vi "DSF.Engine.Execution.Builder.Initialize Intermediate Buffers.vi"(8 "error in (no error)":errorcluster, 11 "Builder in":refnum<class "DSF.Engine.Execution.Builder.lvclass">) -> (0 "error out":errorcluster, 2 "Data Type Buffers":T1, 3 "Builder out":refnum<class "DSF.Engine.Execution.Builder.lvclass">)   [LabVIEW 2016, in "DSF.Engine.lvlib" / "DSF.Engine.Execution.Builder.lvclass"]
uses:
  DSF.Engine.Execution.Builder.lvclass
  DSF.Engine.Execution.Builder.Type Buffers.ctl
  DSF.Engine.Execution.Builder.lvclass/DSF.Engine.Execution.Builder.ctl
  Cache/DSF.Engine.Memory.Cache.Framework.lvclass/DSF.Engine.Memory.Cache.Framework.ctl
  Cache/DSF.Engine.Memory.Cache.Plugin.lvclass/DSF.Engine.Memory.Cache.Plugin.ctl
  Cache/DSF.Engine.Memory.Cache.Transfer.lvclass/DSF.Engine.Memory.Cache.Transfer.ctl
  Cache/DSF.Engine.Memory.Cache.Framework.Get Plugin Caches.vi
  Cache/DSF.Engine.Memory.Cache.Plugin.Get Largest Count.All Types.vi
  Cache/DSF.Engine.Memory.Cache.Plugin.Get Transfer Caches.vi
  Cache/DSF.Engine.Memory.Cache.Transfer.Get Largest Count.All Types.vi
  Cache/DSF.Engine.Memory.Cache.Transfer.Get Channel Configuration.vi
  Cache/DSF.Engine.Memory.Cache.Framework.lvclass
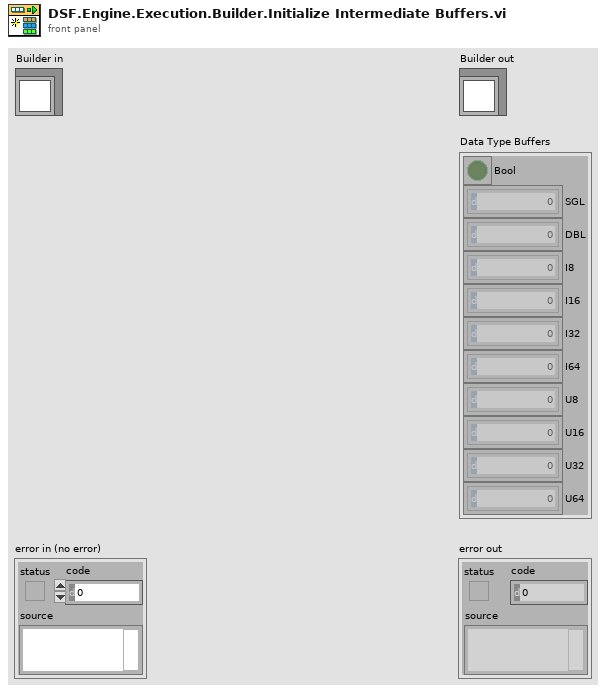
[diagram p1: front panel]
types:
  T1 = typedef "DSF.Engine.lvlib/DSF.Engine.Execution.Builder.lvclass/DSF.Engine.Execution.Builder.Type Buffers.ctl" = cluster{"Bool":bool[], "SGL":sgl[], "DBL":dbl[], "I8":i8[], "I16":i16[], "I32":i32[], "I64":i64[], "U8":u8[], "U16":u16[], "U32":u32[], "U64":u64[]}
  T2 = typedef "DSF.Shared.lvlib/DSF.Shared.Data Type Counts.ctl" = cluster{"Bool":u64, "SGL":u64, "DBL":u64, "I8":u64, "I16":u64, "I32":u64, "I64":u64, "U8":u64, "U16":u64, "U32":u64, "U64":u64}
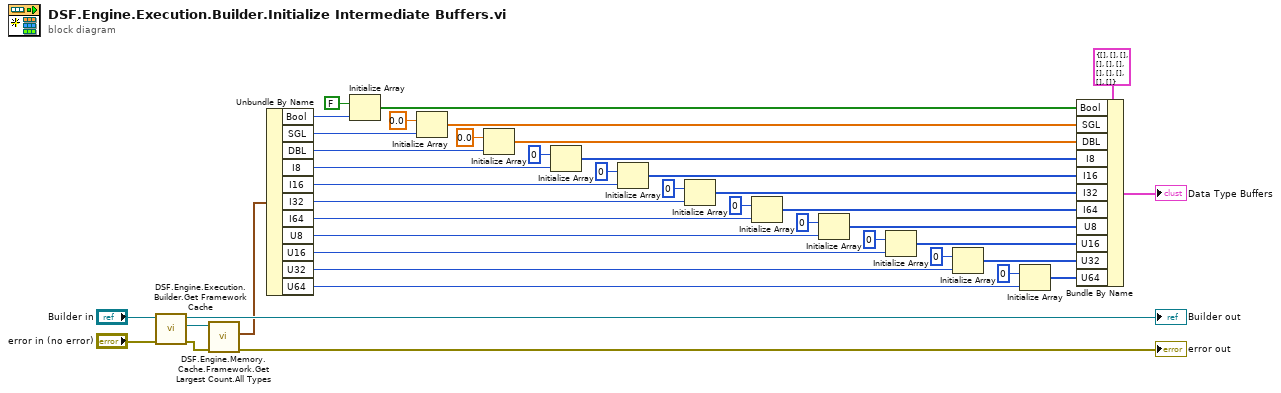
[diagram p0: block diagram]
diagram:
  n1 = call "DSF.Engine.Execution.Builder.Get Framework Cache.vi"("error in (no error)"="error in (no error)", "Builder in"="Builder in") -> ("error out"=w39:errorcluster, "Framework Cache"=w40:refnum<class "DSF.Engine.Memory.Cache.Framework.lvclass">, "Builder out"=→"Builder out":refnum<class "DSF.Engine.Execution.Builder.lvclass">)  [unwired: 7 in]
  n2 = call "DSF.Engine.Memory.Cache.Framework.Get Largest Count.All Types.vi"("error in (no error)"=w39, "Framework Cache in"=w40) -> ("error out"=→"error out":errorcluster, "Data Type Counts out"=w36:T2)  [unwired: 7 in, 1 out]
  n3 = Unbundle By Name(w36) -> ("Bool"=w34:u64, "SGL"=w32:u64, "DBL"=w26:u64, "I8"=w23:u64, "I16"=w15:u64, "I32"=w14:u64, "I64"=w13:u64, "U8"=w12:u64, "U16"=w11:u64, "U32"=w10:u64, "U64"=w9:u64)
  n4 = Initialize Array(FALSE, w34) -> (w30:bool[])
  n5 = Initialize Array(sgl 0.0, w32) -> (w29:sgl[])
  n6 = Initialize Array(0.0, w26) -> (w25:dbl[])
  n7 = Initialize Array(i8 0, w23) -> (w1:i8[])
  n8 = Initialize Array(i16 0, w15) -> (w2:i16[])
  n9 = Initialize Array(0, w14) -> (w3:i32[])
  n10 = Initialize Array(i64 0, w13) -> (w4:i64[])
  n11 = Initialize Array(u8 0, w12) -> (w5:u8[])
  n12 = Initialize Array(u16 0, w11) -> (w6:u16[])
  n13 = Initialize Array(u32 0, w10) -> (w7:u32[])
  n14 = Initialize Array(u64 0, w9) -> (w8:u64[])
  n15 = Bundle By Name(cluster=T1 {"Bool"=[], "SGL"=[], "DBL"=[], "I8"=[], "I16"=[], "I32"=[], "I64"=[], "U8"=[], "U16"=[], "U32"=[], "U64"=[]} ("Data Type Buffers"), "Bool"=w30, "SGL"=w29, "DBL"=w25, "I8"=w1, "I16"=w2, "I32"=w3, "I64"=w4, "U8"=w5, "U16"=w6, "U32"=w7, "U64"=w8) -> (→"Data Type Buffers":T1)
